vi "Reactor Write Client.vi"() -> ()   [LabVIEW 2017]
uses:
  <vilib>/OPCUA/controls/Write Status.ctl
  <vilib>/OPCUA/controls/NodeId.ctl
  <vilib>/OPCUA/client/Multiple Write Double Array.vi
  <vilib>/OPCUA/client/Multiple Write Bool Array.vi
  <vilib>/OPCUA/NI OPC UA Client.lvlib
panel:
  in  "Stop Reactor Digital Control":bool
  in  "Node Status":T1 items=["Good"=0, "Uncertain_InitialValue"=1083310080, "Uncertain_LastUsableValue"=1083179008, "Uncertain_SensorNotAccurate"=1083375616, "Uncertain_EngineeringUnitsExceeded"=1083441152, "Bad_NoCommunication"=2150694912, "Bad_NotReadable"=2151284736, "Bad_NotWritable"=2151350272, "Bad_OutOfRange"=2151415808, "Bad_WaitingForInitialData"=2150760448]
  in  "Time Stamp":timestamp
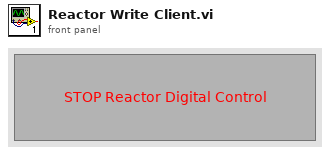
[diagram p1: front panel]
types:
  T1 = typedef "Write Status.ctl" = u32
  T2 = cluster{"message mode":enum16{"None", "Sign", "Sign and Encrypt"}, "security":enum16{"Basic256", "Basic128Rsa15"}}
  T3 = typedef "OPC UA Client Refnum.ctl" = refnum<k21>
  T4 = typedef "NodeId.ctl" = string
  T5 = cluster{"node ID":T4, "value":bool[], "timestamp (current time)":timestamp, "node status":T1}
  T6 = cluster{"node ID":T4, "value":dbl[], "timestamp (current time)":timestamp, "node status":T1}
  T7 = cluster{"node ID":T4, "value":dbl[], "timestamp (current time)":timestamp, "node status":T1}[]
  T8 = cluster{"node ID":T4, "value":bool[], "timestamp (current time)":timestamp, "node status":T1}[]
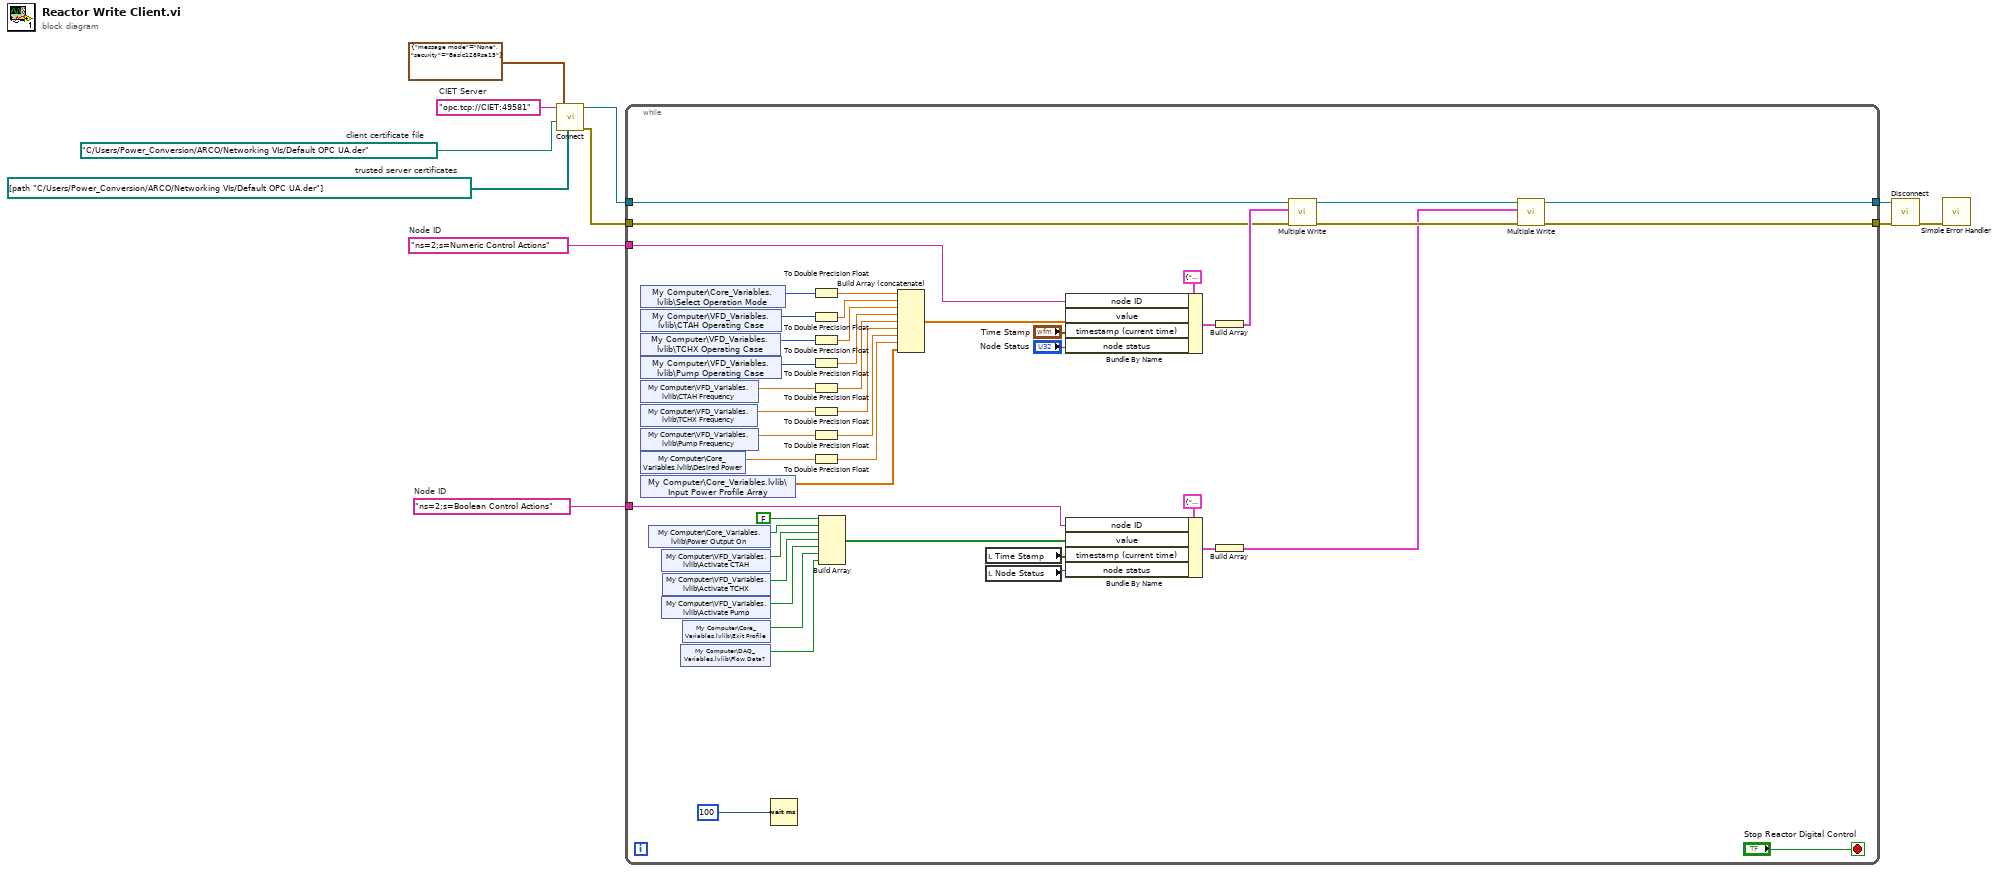
[diagram p0: block diagram]
diagram:
  w4 = "ns=2;s=Boolean Control Actions"  # Node ID
  w5 = "ns=2;s=Numeric Control Actions"  # Node ID
  w8 = path[] [path "C:/Users/Power_Conversion/ARCO/Networking VIs/Default OPC UA.der"]  # trusted server certificates
  w9 = path "C:/Users/Power_Conversion/ARCO/Networking VIs/Default OPC UA.der"  # client certificate file
  w11 = "opc.tcp://CIET:49581"  # CIET Server
  n1 = call <vilib>:"Connect.vi"("trusted server certificates"=w8, "client certificate file"=w9, "security policy"=T2 {"message mode"=enum."None", "security"=enum."Basic128Rsa15"}, "server endpoint URL"=w11) -> ("error out"=w6:errorcluster, "OPC UA client refnum out"=w7:T3)  [unwired: 5 in, 1 out]
  n2 = while {
    tunnel: w7 -> [w38]
    tunnel: w6 -> [w36]
    tunnel: w5 -> [w26]
    tunnel: w4 -> [w25]
    tunnel: [w22] -> w3
    tunnel: [w21] -> w2
    stop <- "Stop Reactor Digital Control" stop-if-true
    n3 = shared-variable "My Computer\\Core_Variables.lvlib\\Select Operation Mode"() -> (w57:u16)  [unwired: 1 in, 1 out]
    n4 = shared-variable "My Computer\\VFD_Variables.lvlib\\CTAH Operating Case"() -> (w54:i32)  [unwired: 1 in, 1 out]
    n5 = shared-variable "My Computer\\VFD_Variables.lvlib\\TCHX Operating Case"() -> (w55:i32)  [unwired: 1 in, 1 out]
    n6 = shared-variable "My Computer\\VFD_Variables.lvlib\\Pump Operating Case"() -> (w56:i32)  [unwired: 1 in, 1 out]
    n7 = shared-variable "My Computer\\VFD_Variables.lvlib\\CTAH Frequency"() -> (w20:sgl)  [unwired: 1 in, 1 out]
    n8 = shared-variable "My Computer\\VFD_Variables.lvlib\\TCHX Frequency"() -> (w19:sgl)  [unwired: 1 in, 1 out]
    n9 = shared-variable "My Computer\\VFD_Variables.lvlib\\Pump Frequency"() -> (w18:sgl)  [unwired: 1 in, 1 out]
    n10 = shared-variable "My Computer\\Core_Variables.lvlib\\Desired Power"() -> (w17:sgl)  [unwired: 1 in, 1 out]
    n11 = shared-variable "My Computer\\Core_Variables.lvlib\\Input Power Profile Array"() -> (w12:dbl[])  [unwired: 1 in, 1 out]
    n12 = shared-variable "My Computer\\Core_Variables.lvlib\\Power Output On"() -> (w48:bool)  [unwired: 1 in, 1 out]
    n13 = shared-variable "My Computer\\VFD_Variables.lvlib\\Activate CTAH"() -> (w47:bool)  [unwired: 1 in, 1 out]
    n14 = shared-variable "My Computer\\VFD_Variables.lvlib\\Activate Pump"() -> (w45:bool)  [unwired: 1 in, 1 out]
    n15 = shared-variable "My Computer\\VFD_Variables.lvlib\\Activate TCHX"() -> (w46:bool)  [unwired: 1 in, 1 out]
    n16 = shared-variable "My Computer\\DAQ_Variables.lvlib\\Flow Data?"() -> (w43:bool)  [unwired: 1 in, 1 out]
    n17 = shared-variable "My Computer\\Core_Variables.lvlib\\Exit Profile"() -> (w44:bool)  [unwired: 1 in, 1 out]
    n18 = Wait (ms)(milliseconds to wait=u32 100) -> ()  [unwired: 1 out]
    n19 = To Double Precision Float(number=w57) -> (double precision float=w53:dbl)
    n20 = To Double Precision Float(number=w54) -> (double precision float=w52:dbl)
    n21 = To Double Precision Float(number=w55) -> (double precision float=w51:dbl)
    n22 = To Double Precision Float(number=w56) -> (double precision float=w50:dbl)
    n23 = To Double Precision Float(number=w20) -> (double precision float=w16:dbl)
    n24 = To Double Precision Float(number=w19) -> (double precision float=w15:dbl)
    n25 = To Double Precision Float(number=w18) -> (double precision float=w14:dbl)
    n26 = To Double Precision Float(number=w17) -> (double precision float=w13:dbl)
    n27 = Build Array(FALSE, w48, w47, w46, w45, w44, w43) -> (w31:bool[])
    n28 = Build Array (concatenate)(w53, w52, w51, w50, w16, w15, w14, w13, w12) -> (w41:dbl[])
    n29 = local read "Time Stamp"() -> (w28:timestamp)
    n30 = local read "Node Status"() -> (w27:T1)
    n31 = Bundle By Name(cluster=T6 {"node ID"="", "value"=[], "timestamp (current time)"=timestamp(0 s since 1904-01-01), "node status"=0} ("request"), "node ID"=w26, "value"=w41, "timestamp (current time)"="Time Stamp", "node status"="Node Status") -> (w40:T6)
    n32 = Bundle By Name(cluster=T5 {"node ID"="", "value"=[], "timestamp (current time)"=timestamp(0 s since 1904-01-01), "node status"=0} ("request"), "node ID"=w25, "value"=w31, "timestamp (current time)"=w28, "node status"=w27) -> (w33:T5)
    n33 = Build Array(w40) -> (w39:T7)
    n34 = Build Array(w33) -> (w32:T8)
    n35 = call-poly <vilib>:"Multiple Write.vi"("error in (no error)"=w36, "requests"=w39, "OPC UA client refnum in"=w38) -> ("error out"=w35:errorcluster, "OPC UA client refnum out"=w37:T3)  [unwired: 5 in, 2 out]
    n36 = call-poly <vilib>:"Multiple Write.vi"("error in (no error)"=w35, "requests"=w32, "OPC UA client refnum in"=w37) -> ("error out"=w21:errorcluster, "OPC UA client refnum out"=w22:T3)  [unwired: 5 in, 2 out]
  }
  n37 = call <vilib>:"Disconnect.vi"("error in (no error)"=w2, "OPC UA client refnum in"=w3) -> ("error out"=w1:errorcluster)  [unwired: 9 in]
  n38 = call <vilib>:"Simple Error Handler.vi"("error in (no error)"=w1) -> ()  [unwired: 4 in, 5 out]
